vi "plot -- make visible.vi"(6 "Active Plot":u32, 11 "reference":refnum<vi>) -> (3 "reference out":refnum<vi>)   [LabVIEW 2021]
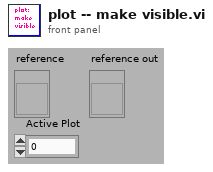
[diagram p1: front panel]
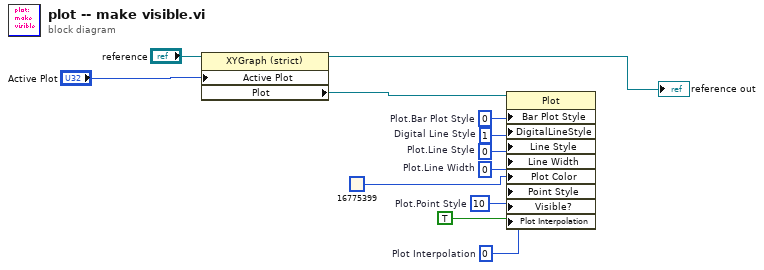
[diagram p0: block diagram]
diagram:
  w5 = u8 10  # Plot.Point Style
  w7 = u8 0  # Plot Interpolation
  w12 = u8 1  # Digital Line Style
  w11 = u8 0  # Plot.Line Width
  w10 = u8 0  # Plot.Line Style
  w9 = u8 0  # Plot.Bar Plot Style
  n1 = property on="Property Node" class="XYGraph (strict)"(reference="reference", "Active Plot"="Active Plot") -> (reference out=→"reference out":refnum<vi>, "Plot"=w8:refnum<vi>)  [unwired: 1 in, 1 out]
  n2 = property class="Plot"(reference=w8, "Bar Plot Style"=w9, "DigitalLineStyle"=w12, "Line Style"=w10, "Line Width"=w11, "Plot Color"=u32 16775399, "Point Style"=w5, "Visible?"=TRUE, "Plot Interpolation"=w7) -> ()  [unwired: 1 in, 2 out]
